vi "Set Error Code.vi"(9 "offset":i32, 10 "code":i32, 11 "error in":errorcluster) -> (1 "offset":i32, 3 "error out":errorcluster)   [LabVIEW 2020, in "Static Errors.lvlib"]
doc: "Sets the code of <b>error</b>."
uses:
  Static Errors.lvlib
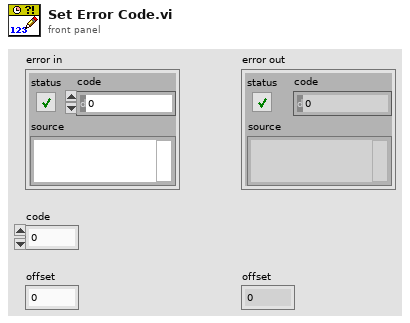
[diagram p1: front panel]
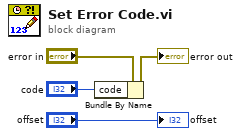
[diagram p0: block diagram]
diagram:
  n1 = Bundle By Name(cluster="error in", "code"="code") -> (→"error out":errorcluster)
  "offset" <- "offset"
